vi "Global Variable Monitor.vi"() -> ()   [LabVIEW 2018, in "Ismatec 4308.lvlib"]
uses:
  Ismatec 78001/Ismatec 4308.lvlib
  Ismatec 78001/Ismatec 4083 Global.ctl
  Ismatec 78001/Ismatec 4083 Global Element.ctl
panel:
  in  "stop 2":bool
  out "Ismatec 78001 Global":T1(array[cluster])
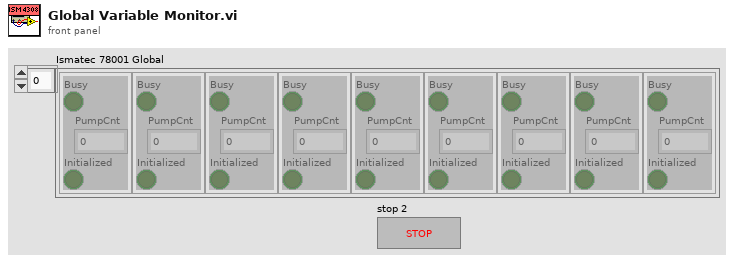
[diagram p1: front panel]
types:
  T1 = cluster{"Busy":bool, "PumpCnt":dbl, "Initialized":bool}[]
  T2 = typedef "Ismatec 4308.lvlib/Ismatec 4083 Global.ctl" = T3[]
  T3 = typedef "Ismatec 4308.lvlib/Ismatec 4083 Global Element.ctl" = cluster{"Busy":bool, "ChannelCnt":dbl, "Initialized":bool, "Current Channel":dbl, "Initialized Channels":dbl[]}
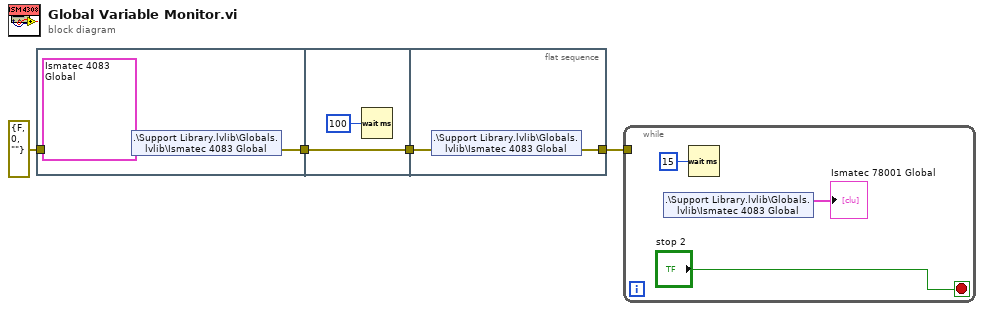
[diagram p0: block diagram]
diagram:
  n1 = flat-sequence {
    tunnel: [w7] -> w4
    tunnel: errorcluster {"status"=FALSE, "code"=0, "source"=""} ("error in (no error)") -> [w6]
    tunnel: w4 -> [w9]
    tunnel: [w9] -> w3
    tunnel: w3 -> [w11]
    tunnel: [w10] -> w2
    frame #0 {
      n2 = shared-variable ".\\Support Library.lvlib\\Globals.lvlib\\Ismatec 4083 Global"(T2 [{"Busy"=FALSE, "ChannelCnt"=0.0, "Initialized"=FALSE, "Current Channel"=0.0, "Initialized Channels"=[]}, {"Busy"=FALSE, "ChannelCnt"=0.0, "Initialized"=FALSE, "Current Channel"=0.0, "Initialized Channels"=[]}, {"Busy"=FALSE, "ChannelCnt"=0.0, "Initialized"=FALSE, "Current Channel"=0.0, "Initialized Channels"=[]}, {"Busy"=FALSE, "ChannelCnt"=0.0, "Initialized"=FALSE, "Current Channel"=0.0, "Initialized Channels"=[]}, {"Busy"=FALSE, "ChannelCnt"=0.0, "Initialized"=FALSE, "Current Channel"=0.0, "Initialized Channels"=[]}, {"Busy"=FALSE, "ChannelCnt"=0.0, "Initialized"=FALSE, "Current Channel"=0.0, "Initialized Channels"=[]}, {"Busy"=FALSE, "ChannelCnt"=0.0, "Initialized"=FALSE, "Current Channel"=0.0, "Initialized Channels"=[]}, {"Busy"=FALSE, "ChannelCnt"=0.0, "Initialized"=FALSE, "Current Channel"=0.0, "Initialized Channels"=[]}, {"Busy"=FALSE, "ChannelCnt"=0.0, "Initialized"=FALSE, "Current Channel"=0.0, "Initialized Channels"=[]}, {"Busy"=FALSE, "ChannelCnt"=0.0, "Initialized"=FALSE, "Current Channel"=0.0, "Initialized Channels"=[]}, {"Busy"=FALSE, "ChannelCnt"=0.0, "Initialized"=FALSE, "Current Channel"=0.0, "Initialized Channels"=[]}, {"Busy"=FALSE, "ChannelCnt"=0.0, "Initialized"=FALSE, "Current Channel"=0.0, "Initialized Channels"=[]}, {"Busy"=FALSE, "ChannelCnt"=0.0, "Initialized"=FALSE, "Current Channel"=0.0, "Initialized Channels"=[]}, {"Busy"=FALSE, "ChannelCnt"=0.0, "Initialized"=FALSE, "Current Channel"=0.0, "Initialized Channels"=[]}, {"Busy"=FALSE, "ChannelCnt"=0.0, "Initialized"=FALSE, "Current Channel"=0.0, "Initialized Channels"=[]}, {"Busy"=FALSE, "ChannelCnt"=0.0, "Initialized"=FALSE, "Current Channel"=0.0, "Initialized Channels"=[]}, {"Busy"=FALSE, "ChannelCnt"=0.0, "Initialized"=FALSE, "Current Channel"=0.0, "Initialized Channels"=[]}, {"Busy"=FALSE, "ChannelCnt"=0.0, "Initialized"=FALSE, "Current Channel"=0.0, "Initialized Channels"=[]}, {"Busy"=FALSE, "ChannelCnt"=0.0, "Initialized"=FALSE, "Current Channel"=0.0, "Initialized Channels"=[]}, {"Busy"=FALSE, "ChannelCnt"=0.0, "Initialized"=FALSE, "Current Channel"=0.0, "Initialized Channels"=[]}, {"Busy"=FALSE, "ChannelCnt"=0.0, "Initialized"=FALSE, "Current Channel"=0.0, "Initialized Channels"=[]}] ("Array"), error in=w6) -> (error out=w7:errorcluster)
    }
    frame #1 {
      n3 = Wait (ms)(milliseconds to wait=u32 100) -> ()  [unwired: 1 out]
    }
    frame #2 {
      n4 = shared-variable ".\\Support Library.lvlib\\Globals.lvlib\\Ismatec 4083 Global"(error in=w11) -> (error out=w10:errorcluster)  [unwired: 1 out]
    }
  }
  n5 = while {
    tunnel: w2 -> [_]
    stop <- "stop 2" stop-if-true
    n6 = shared-variable ".\\Support Library.lvlib\\Globals.lvlib\\Ismatec 4083 Global"() -> (→"Ismatec 78001 Global":T2)  [unwired: 1 in, 1 out]
    n7 = Wait (ms)(milliseconds to wait=u32 15) -> ()  [unwired: 1 out]
  }
